vi "Cursor Redraw Read.vi"(4 "error in (no error)":errorcluster, 6 "Container State":T4, 7 "Display State In":T1={"Numeric"=0.0, "Timeline Ref"=refnum, "Waveform Ref"=refnum, "Fill Plots"=FALSE, "Cursor Redraw"=TRUE}) -> (0 "error out":errorcluster, 2 "Value":bool, 3 "Display State Out":T1={"Numeric"=0.0, "Timeline Ref"=refnum, "Waveform Ref"=refnum, "Fill Plots"=FALSE, "Cursor Redraw"=TRUE})   [LabVIEW 2013, in "XGrapher.xctl"]
uses:
  XGrapher.xctl
  <vilib>/_xctls/Container State.ctl
  State 1.ctl
  Typedefs/Xctrl-Timeline graph ref.ctl
  Typedefs/Xctrl-Waveform graph ref.ctl
  <vilib>/_xctls/XControlSupport.lvlib
panel:
  # "Replace the Value Indicator below with an Indicator of desired type.\nDo not remove this Indicator or the others from the connector pane. \nDo not change the connector pane pattern.\nThe Value Indicator should always be the second terminal from top on the output side in the connector pane."
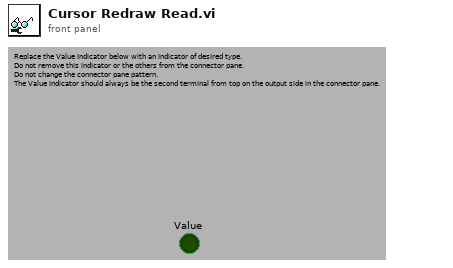
[diagram p1: front panel]
types:
  T1 = typedef "XGrapher.xctl/State 1.ctl" = cluster{"Numeric":dbl, "Timeline Ref":T2, "Waveform Ref":T3, "Fill Plots":bool, "Cursor Redraw":bool}
  T2 = typedef "XGrapher.xctl/Xctrl-Timeline graph ref.ctl" = refnum<vi>
  T3 = typedef "XGrapher.xctl/Xctrl-Waveform graph ref.ctl" = refnum<vi>
  T4 = typedef "XControlSupport.lvlib/Container State.ctl" = cluster{"Indicator?":bool, "Run Mode?":bool, " Refnum":refnum<vi>}
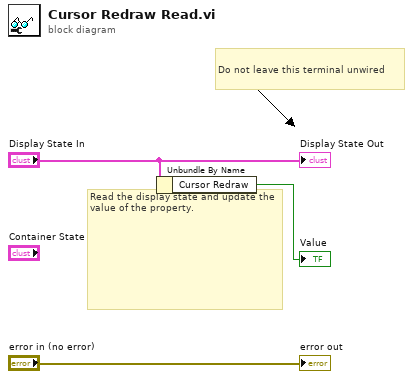
[diagram p0: block diagram]
diagram:
  # "Do not leave this terminal unwired"
  # "Read the display state and update the value of the property."
  n1 = Unbundle By Name("Display State In") -> ("Cursor Redraw"=→"Value":bool)
  "error out" <- "error in (no error)"
  "Display State Out" <- "Display State In"
